vi "Multidot T1 measurements.vi"() -> ()   [LabVIEW 2012]
uses:
  <vilib>/Utility/file.llb/Write To Spreadsheet File (DBL).vi
panel:
  in  "Y Parameters":T1={"Number of Y Steps"=200, "Max Y (V)"=2.0, "Min Y (V)"=-2.0}
  in  "X":T2={"Number of X Steps"=200, "Max X (V)"=2.0, "Min X (V)"=-2.0}
  out "Tracking Loop":dbl=6.0
  in  "N Loop":i32=25000
  in  "ref?":bool=TRUE
  in  "Sig/Ref pause":dbl=3e-07
  in  "APD signal width":dbl=3e-07
  in  "AOM Pulse length":dbl=2.5e-06
  in  "Signal delay":dbl=1.16e-06
  in  "AOM Rest time":dbl=2e-08
  in  "Path to spinapi.dll":path=path "C:/SpinCore/SpinAPI/dll/spinapi64.dll"
  in  "Rest time No. Steps":i32=20
  in  "Rest time Max":dbl=0.0002
  in  "Rest time Min":dbl=2e-08
  in  "type":u16(ring)=1 items=["Linear", "Logarithmic"]
  in  "Scan Interval (sec)":dbl=2.0
  in  "Collection Time (sec)":dbl=3.0
  in  "File Path Control":path
  in  "Array - Numeric":dbl[][](array[numeric])=[[0.0, 0.0], [0.0, 0.0], [0.0, 0.0], [0.0, 0.0], [0.0, 0.0], [0.0, 0.0]]
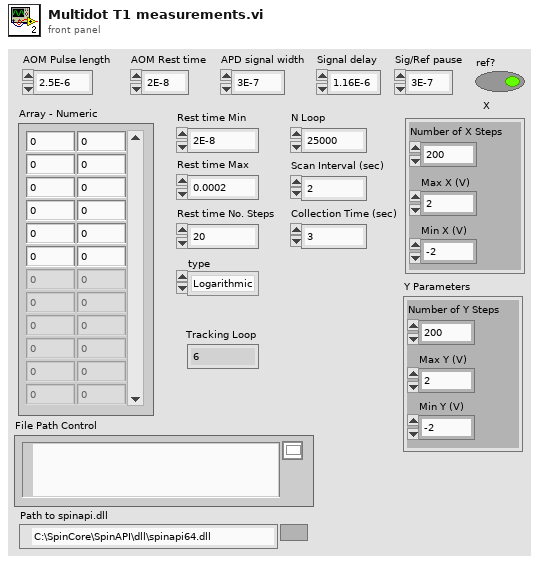
[diagram p1: front panel]
types:
  T1 = cluster{"Number of Y Steps":i32, "Max Y (V)":dbl, "Min Y (V)":dbl}
  T2 = cluster{"Number of X Steps":i32, "Max X (V)":dbl, "Min X (V)":dbl}
  T3 = enum16{"Stop", "Track", "EPR", "Load Pulse Sequence"}
  T4 = cluster{"Instruct Data":i32, "Op Code":i32, "Flags":bool[], "Comments":string, "Time (s)":dbl}
  T5 = enum16{"Pulse Program", "Frequency Registers", "TX Phase Registers", "RX Phase Registers"}
  T6 = cluster{"Instruct Data":i32, "Op Code":i32, "Flags":bool[], "Comments":string, "Time (s)":dbl}[]
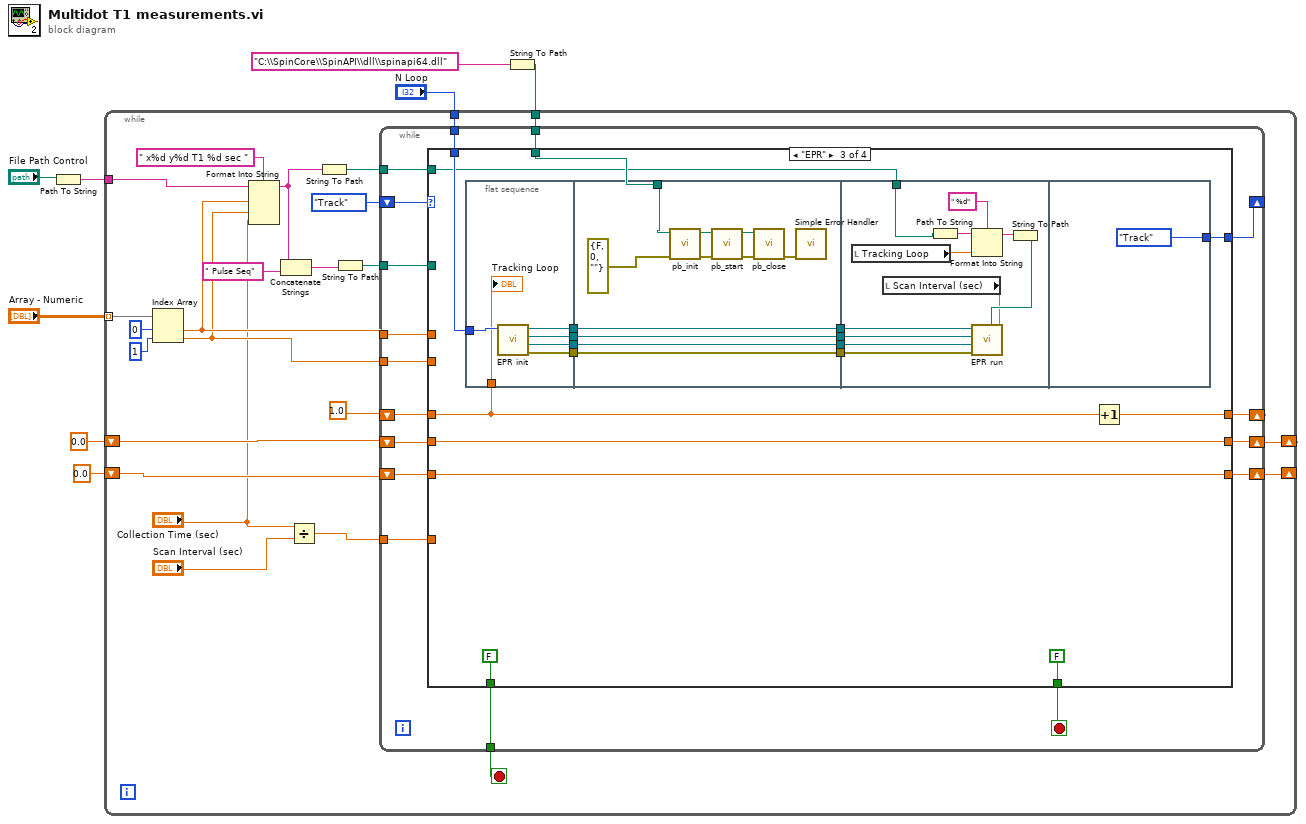
[diagram p0: block diagram]
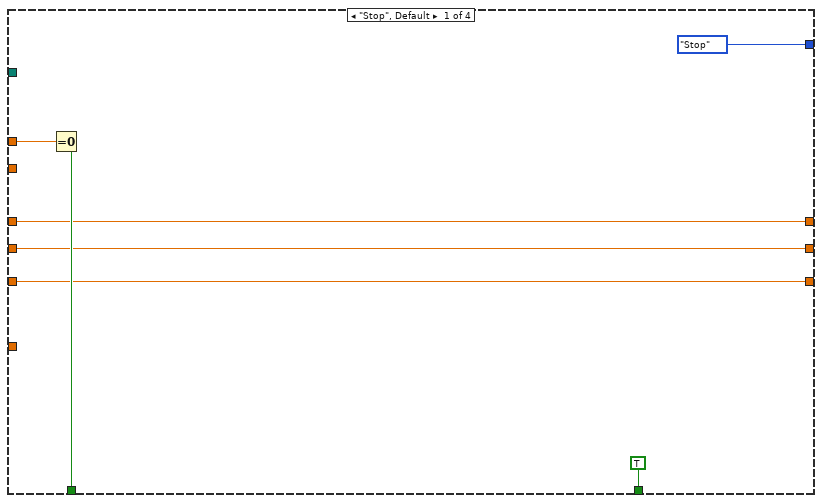
[diagram p2: hidden frame]
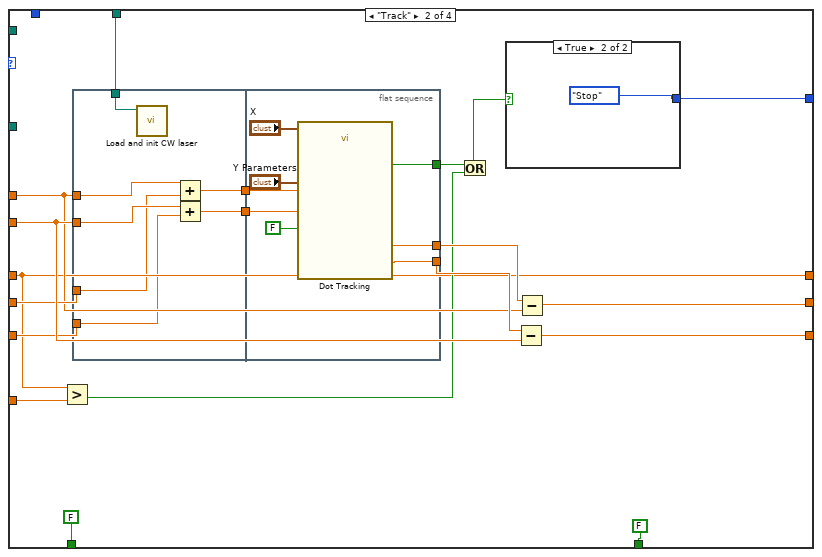
[diagram p3: hidden frame]
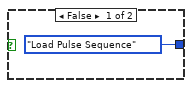
[diagram p4: hidden frame]
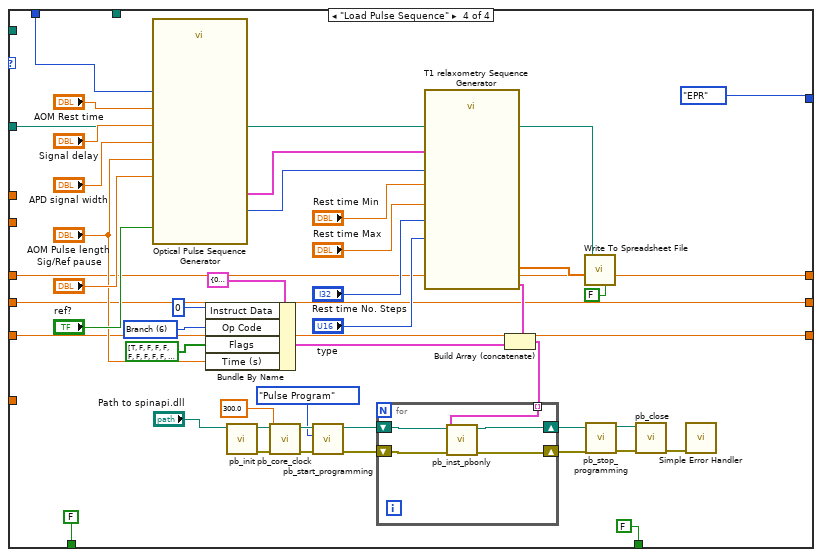
[diagram p5: hidden frame]
diagram:
  n1 = Path To String(path="File Path Control") -> (string=w5:string)
  n2 = String To Path(string="C:\\SpinCore\\SpinAPI\\dll\\spinapi64.dll") -> (path=w2:path)
  n3 = while {
    tunnel: "Array - Numeric" -> [w32] mode=indexing
    shift-right: [w24] -> _
    shift-left: 0.0 -> [w20]
    shift-right: [w23] -> _
    shift-left: 0.0 -> [w22]
    tunnel: w5 -> [w29]
    tunnel: w2 -> [w26]
    tunnel: "N Loop" -> [w18]
    stop <- w13 stop-if-true
    n4 = Index Array(array=w32, index #1=0 ("index"), index #2=1 ("index")) -> (element #1=w21:dbl, element #2=w19:dbl)
    n5 = Format Into String(format string=" x%d y%d T1 %d sec ", initial string=w29, w21, w19, "Collection Time (sec)") -> (resulting string=w17:string)  [unwired: 1 in, 1 out]
    n6 = Concatenate Strings(w17, " Pulse Seq" ("string")) -> (w15:string)
    n7 = Divide(x="Collection Time (sec)", y="Scan Interval (sec)") -> (x/y=w10:dbl)
    n8 = String To Path(string=w17) -> (path=w16:path)
    n9 = String To Path(string=w15) -> (path=w14:path)
    n10 = while {
      tunnel: w19 -> [w47]
      tunnel: w21 -> [w48]
      tunnel: w26 -> [w49]
      shift-right: [w45] -> w24
      shift-left: w20 -> [w44]
      shift-right: [w46] -> w23
      shift-left: w22 -> [w43]
      shift-right: [w40] -> _
      shift-left: T3."Track" -> [w42]
      tunnel: w18 -> [w39]
      tunnel: w16 -> [w38]
      tunnel: w14 -> [w37]
      shift-right: [w35] -> _
      shift-left: 1.0 -> [w36]
      tunnel: [w34] -> w13
      tunnel: w10 -> [w33]
      stop <- w41 stop-if-true
      n11 = case shown="\"EPR\"" w42 {
        tunnel: w49 -> [_ w75 w102 _]
        tunnel: w48 -> [w55 w68 _ _]
        tunnel: w47 -> [_ w71 _ _]
        tunnel: [w51 w74 w99 w142] -> w45
        tunnel: [w50 w57 w95 w141] -> w46
        tunnel: w44 -> [w51 w70 w99 w142]
        tunnel: w43 -> [w50 w69 w95 w141]
        tunnel: [T3."Stop" w64 w96 T3."EPR"] -> w40
        tunnel: [TRUE FALSE FALSE FALSE] -> w41
        tunnel: w39 -> [_ _ w101 w146]
        tunnel: w38 -> [_ _ w100 _]
        tunnel: w37 -> [_ _ _ w145]
        tunnel: w36 -> [w52 w58 w93 w143]
        tunnel: [w52 w58 w97 w143] -> w35
        tunnel: [w54 FALSE FALSE FALSE] -> w34
        tunnel: w33 -> [_ w61 _ _]
        frame "Stop", Default {
          n12 = Equal To 0?(x=w55) -> (x = 0?=w54:bool)
        }
        frame "Track" {
          n13 = Greater?(x=w58, y=w61) -> (0:w59:bool)
          n14 = flat-sequence {
            tunnel: w75 -> [w84]
            tunnel: w68 -> [w83]
            tunnel: w71 -> [w82]
            tunnel: w70 -> [w81]
            tunnel: w69 -> [w80]
            tunnel: [w79] -> w67
            tunnel: [w78] -> w66
            tunnel: [w92] -> w73
            tunnel: [w91] -> w72
            tunnel: w67 -> [w90]
            tunnel: w66 -> [w89]
            tunnel: [w87] -> w65
            frame #0 {
              n15 = call "Load and init CW laser.vi"("path in"=w84) -> ()  [unwired: 11 in]
              n16 = Add(x=w83, y=w81) -> (x+y=w79:dbl)
              n17 = Add(x=w82, y=w80) -> (x+y=w78:dbl)
            }
            frame #1 {
              n18 = call "Dot Tracking.vi"("X"="X", "Y Parameters"="Y Parameters", "X Pos"=w90, "Y pos"=w89, "Z-track?"=FALSE) -> ("X Position"=w92:dbl, "Y Position"=w91:dbl, "Gave up?"=w87:bool)  [unwired: 4 in, 4 out]
            }
          }
          n19 = Or(x=w65, y=w59) -> (x .or. y?=w60:bool)
          n20 = case shown="True" w60 {
            tunnel: [T3."Load Pulse Sequence" T3."Stop"] -> w64
            frame False {
            }
            frame True {
            }
          }
          n21 = Subtract(x=w72, y=w71) -> (x-y=w57:dbl)
          n22 = Subtract(x=w73, y=w68) -> (x-y=w74:dbl)
        }
        frame "EPR" {
          n23 = flat-sequence {
            tunnel: [w116] -> w110
            tunnel: [w115] -> w109
            tunnel: [w114] -> w108
            tunnel: [w113] -> w107
            tunnel: w101 -> [w112]
            tunnel: w93 -> [w111]
            tunnel: [w121] -> w106
            tunnel: w110 -> [w121]
            tunnel: [w120] -> w105
            tunnel: w109 -> [w120]
            tunnel: [w119] -> w104
            tunnel: w108 -> [w119]
            tunnel: [w118] -> w103
            tunnel: w107 -> [w118]
            tunnel: w102 -> [w117]
            tunnel: w106 -> [w132]
            tunnel: w105 -> [w131]
            tunnel: w104 -> [w130]
            tunnel: w103 -> [w129]
            tunnel: w100 -> [w128]
            tunnel: [T3."Track"] -> w96
            frame #0 {
              n24 = call "EPR init.vi"("N loops"=w112) -> ("error out"=w113:errorcluster, "ref task out"=w114:refnum<k21>, "sig task out"=w115:refnum<k21>, "clock task out"=w116:refnum<k21>)  [unwired: 7 in]
              "Tracking Loop" <- w111
            }
            frame #1 {
              n25 = call "pb_init.vi"("error in (no error)"=errorcluster {"status"=FALSE, "code"=0, "source"=""}, "path in"=w117) -> ("error out"=w125:errorcluster, "path out"=w123:path)  [unwired: 1 in, 7 out]
              n26 = call "pb_start.vi"("error in (no error)"=w125, "path in"=w123) -> ("error out"=w126:errorcluster, "path out"=w122:path)  [unwired: 1 in, 7 out]
              n27 = call "pb_close.vi"("error in (no error)"=w126, "path in"=w122) -> ("error out"=w127:errorcluster)  [unwired: 9 out]
              n28 = call <vilib>:"Simple Error Handler.vi"("error in (no error)"=w127) -> ()  [unwired: 1 in, 8 out]
            }
            frame #2 {
              n29 = local read "Tracking Loop"() -> (w135:dbl)
              n30 = local read "Scan Interval (sec)"() -> (w133:dbl)
              n31 = Path To String(path=w128) -> (string=w137:string)
              n32 = Format Into String(format string=" %d", initial string=w137, w135) -> (resulting string=w136:string)  [unwired: 1 in, 1 out]
              n33 = String To Path(string=w136) -> (path=w134:path)
              n34 = call "EPR run.vi"("control task in"=w132, "sig task in"=w131, "ref task in"=w130, "error in"=w129, "file path (dialog if empty)"=w134, "Measurement Interval"=w133) -> ()  [unwired: 4 in]
            }
            frame #3 {
            }
          }
          n35 = Increment(x=w93) -> (x+1=w97:dbl)
        }
        frame "Load Pulse Sequence" {
          w176 = 6 items=["Continue", "Stop", "Loop", "End Loop", "JSR", "RTS", "Branch", "Long Delay", "Wait"] ("Op Code")
          n36 = call "Optical Pulse Sequence Generator.vi"("ref?"="ref?", "N Loop"=w146, "Sig/Ref pause"="Sig/Ref pause", "AOM Rest time"="AOM Rest time", "Signal delay"="Signal delay", "APD signal width"="APD signal width", "AOM Pulse length"="AOM Pulse length") -> ("Array"=w157:T6, "No. Instructions"=w156:i32)  [unwired: 3 in]
          n37 = Bundle By Name(cluster=T4 {"Instruct Data"=0, "Op Code"=0, "Flags"=[FALSE, FALSE, FALSE, FALSE, FALSE, FALSE, FALSE, FALSE, FALSE, FALSE, FALSE, FALSE, FALSE, FALSE, FALSE, FALSE, FALSE, FALSE, FALSE, FALSE, FALSE, TRUE, TRUE, TRUE], "Comments"="", "Time (s)"=0.01} ("PB Inst 2"), "Instruct Data"=0, "Op Code"=w176, "Flags"=bool[] [TRUE, FALSE, FALSE, FALSE, FALSE, FALSE, FALSE, FALSE, FALSE, FALSE, FALSE, FALSE, FALSE, FALSE, FALSE, FALSE, FALSE, FALSE, FALSE, FALSE, FALSE, TRUE, TRUE, TRUE], "Time (s)"="AOM Pulse length") -> (w150:T4)
          n38 = call "pb_init.vi"("path in"="Path to spinapi.dll") -> ("error out"=w165:errorcluster, "path out"=w163:path)  [unwired: 3 in, 6 out]
          n39 = call "pb_core_clock.vi"("error in (no error)"=w165, "clock_freq (MHz)"=300.0, "path in"=w163) -> ("error out"=w166:errorcluster, "path out"=w164:path)  [unwired: 7 in]
          n40 = call "pb_start_programming.vi"("error in (no error)"=w166, "Device"=T5."Pulse Program", "path in"=w164) -> ("error out"=w169:errorcluster, "path out"=w168:path)  [unwired: 1 in, 6 out]
          n41 = call "T1 relaxometry Sequence Generator.vi"("Optical Pulse"=w157, "No. Instructions"=w156, "type"="type", "Rest time No. Steps"="Rest time No. Steps", "Rest time Max"="Rest time Max", "Rest time Min"="Rest time Min") -> ("Pulse Width"=w148:dbl[], "Pulse Sequence Out"=w151:T6)  [unwired: 4 in]
          n42 = Build Array (concatenate)(w151, w150) -> (w149:T6)
          n43 = for {
            shift-right: [w185] -> w170
            shift-left: w168 -> [w187]
            shift-right: [w184] -> w171
            shift-left: w169 -> [w186]
            tunnel: w149 -> [w183] mode=indexing
            n44 = call "pb_inst_pbonly.vi"("error in (no error)"=w186, "PB Instruction"=w183, "path in"=w187) -> ("error out"=w184:errorcluster, "path out"=w185:path)  [unwired: 2 in, 5 out]
          }
          n45 = call-poly <vilib>:"Write To Spreadsheet File.vi"("transpose? (no:F)"=FALSE, "1D data"=w148, "file path (dialog if empty)"=w145) -> ()  [unwired: 5 in, 1 out]
          n46 = call "pb_stop_programming.vi"("error in (no error)"=w171, "path in"=w170) -> ("error out"=w162:errorcluster, "path out"=w161:path)  [unwired: 1 in, 7 out]
          n47 = call "pb_close.vi"("error in (no error)"=w162, "path in"=w161) -> ("error out"=w173:errorcluster)  [unwired: 9 out]
          n48 = call <vilib>:"Simple Error Handler.vi"("error in (no error)"=w173) -> ()  [unwired: 1 in, 8 out]
        }
      }
    }
  }
